vi "Wait_ErrorCluster.vi"(8 "error in":errorcluster, 11 "milliseconds to wait":u32) -> (0 "error out":errorcluster)   [LabVIEW 2022 SP3, in "hse-misc.lvlib"]
doc: "Simple wrapper for the Wait function that allows for data flow.\n\n\n\n____\nHAMPEL SOFTWARE ENGINEERING v3.8.0 (2023-12-18 14:41)"
uses:
  hse-misc.lvlib
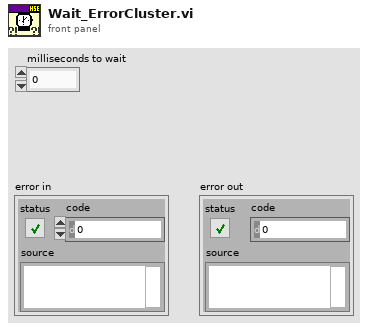
[diagram p1: front panel]
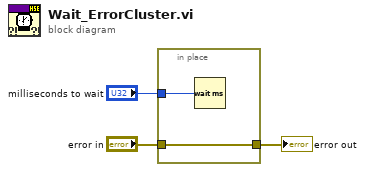
[diagram p0: block diagram]
diagram:
  n1 = in-place {
    in-place-border: "error in" -> [w5]
    in-place-border: [w5] -> w3
    in-place-border: "milliseconds to wait" -> [w4]
    n2 = Wait (ms)(milliseconds to wait=w4) -> ()  [unwired: 1 out]
  }
  "error out" <- w3
